vi "Set Default Static Document.vi"(8 "error in (no error)":errorcluster, 9 "Privilege Mapping":T1(array[cluster]), 10 "Default static document":string, 11 "NI_AB_API_RESTful in":refnum<class "NI_AB_API_RESTful.lvclass">) -> (0 "error out":errorcluster, 3 "NI_AB_API_RESTful out":refnum<class "NI_AB_API_RESTful.lvclass">)   [LabVIEW 2020, in "NI_AB_API_RESTful.lvclass"]
uses:
  <vilib>/AppBuilder/AB_API/RESTful/NI_AB_API_RESTful.lvclass
  <vilib>/AppBuilder/AB_API/RESTful/NI_AB_API_RESTful.lvclass/NI_AB_API_RESTful.ctl
  <vilib>/AppBuilder/AB_API/Build/NI_AB_API_Build.lvclass
  <vilib>/AppBuilder/AB_Classes/RESTful/AB_RESTfulWebService.lvclass
  e:/builds/penguin/labview/branches/2020/dev/dist/vi.lib/AppBuilder/AB_API/Targetfile/NI_AB_API_Targetfile.lvclass
  e:/builds/penguin/labview/branches/2020/dev/dist/vi.lib/AppBuilder/AB_API/Build/NI_AB_API_Build.lvclass
  e:/builds/penguin/labview/branches/2020/dev/dist/vi.lib/AppBuilder/AB_API/RESTful/NI_AB_API_RESTful.lvclass
  e:/builds/penguin/labview/branches/2020/dev/dist/vi.lib/AppBuilder/AB_Classes/WebService/AB_WebService.lvclass
  e:/builds/penguin/labview/branches/2020/dev/dist/vi.lib/AppBuilder/AB_Classes/TargetFile/AB_Targetfile.lvclass
  e:/builds/penguin/labview/branches/2020/dev/dist/vi.lib/AppBuilder/AB_Classes/Build/AB_Build.lvclass
  e:/builds/penguin/labview/branches/2020/dev/dist/vi.lib/AppBuilder/AB_Classes/RESTful/AB_RESTfulWebService.lvclass
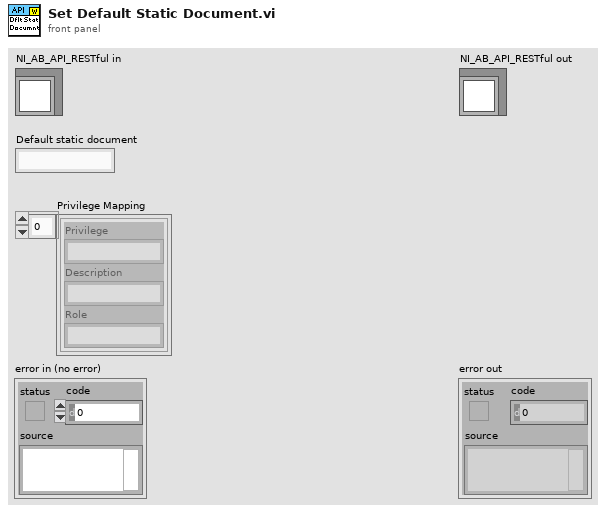
[diagram p1: front panel]
types:
  T1 = cluster{"Privilege":string, "Description":string, "Role":string}[]
  T2 = typedef "AB_RESTfulWebService.ctl" = cluster{"routing templates":T3[], "defaultStaticDoc":string, "eng_attributes":T6[], "Privilege Mapping":cluster{"Privilege":string, "Description":string, "Role":string}[]}
  T3 = typedef "AB_RESTful_RoutingTemplate.ctl" = cluster{"Template":string, "Routing Type":T4, "HTTP Method Type":T5, "VIName":string, "Default String":string, "Require API key":bool, "Auth permissions":string[], "eng_Static Alias":string, "Required Privilege":string}
  T4 = typedef "AB_RESTful_RoutingType.ctl" = enum32{"Method", "Static"}
  T5 = typedef "AB_RESTful_HTTPMethodType.ctl" = enum32{"GET", "POST", "PUT", "DELETE"}
  T6 = typedef "AB_RESTful_ServiceAttribute.ctl" = cluster{"Name":string, "Service Attribute Type":T7, "Value":string}
  T7 = typedef "AB_RESTful_ServiceAttributeType.ctl" = enum32{"String", "Path"}
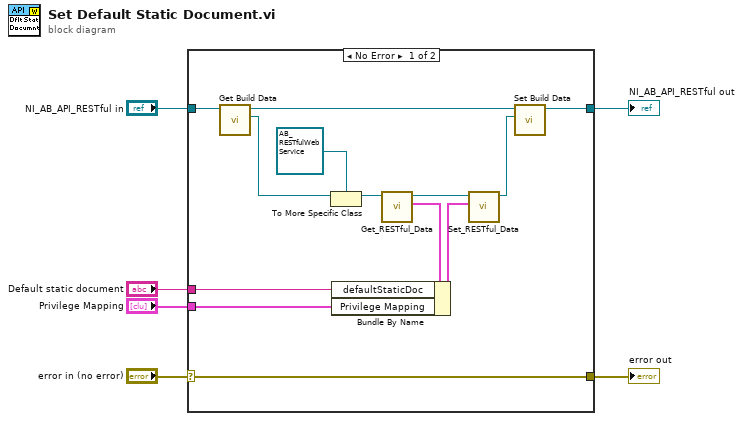
[diagram p0: block diagram]
diagram:
  n1 = case shown="No Error" "error in (no error)" {
    selector: "error in (no error)" -> [w19 w21]
    tunnel: [w19 w21] -> w5
    tunnel: [w16 w20] -> w3
    tunnel: "NI_AB_API_RESTful in" -> [w18 w20]
    tunnel: "Default static document" -> [w8 _]
    tunnel: "Privilege Mapping" -> [w7 _]
    frame No Error {
      n2 = call <vilib>:"Get Build Data.vi"("NI_AB_API_Build in"=w18) -> ("AB_Build.lvclass"=w14:refnum<class "AB_Build.lvclass">, "NI_AB_API_Build out"=w17:refnum<class "NI_AB_API_RESTful.lvclass">)  [unwired: 8 in, 1 out]
      n3 = To More Specific Class(target class=refnum<class "AB_RESTfulWebService.lvclass"> refnum ("AB_RESTfulWebService.lvclass"), reference=w14) -> (specific class reference=w13:refnum<class "AB_RESTfulWebService.lvclass">)  [unwired: 1 in, 1 out]
      n4 = call <vilib>:"Get_RESTful_Data.vi"("Class in"=w13) -> ("data"=w10:T2, "Class out"=w12:refnum<class "AB_RESTfulWebService.lvclass">)  [unwired: 8 in, 1 out]
      n5 = Bundle By Name(cluster=w10, "defaultStaticDoc"=w8, "Privilege Mapping"=w7) -> (w9:T2)
      n6 = call <vilib>:"Set_RESTful_Data.vi"("data"=w9, "Class in"=w12) -> ("Class out"=w11:refnum<class "AB_RESTfulWebService.lvclass">)  [unwired: 8 in, 1 out]
      n7 = call <vilib>:"Set Build Data.vi"("AB_Build.lvclass"=w11, "NI_AB_API_Build in"=w17) -> ("NI_AB_API_Build out"=w16:refnum<class "NI_AB_API_RESTful.lvclass">)  [unwired: 8 in, 1 out]
    }
    frame Error {
    }
  }
  "error out" <- w5
  "NI_AB_API_RESTful out" <- w3
